vi "Edit_Channel_Panel.vi"(0 "All Channel names":string[](array[string])=["30-10-03:New:Channel new5"], 9 "Result files to read":path[](array[path]), 11 "Selected Row":i32) -> (3 "New Values Out":string[](array[string])=["Test data5"], 4 "New Chs Out":string[](array[string])=["30-10-03:New:Channel new5"], 6 "Cancel Out":bool, 8 "Edit Raw Data Header Info Out":bool, 10 "Plotted rows only?":bool, 12 "Selected Row?":bool, 13 "Edit Raw data files?":bool, 14 "Raw data files in Orig Positions?":bool, 15 "Mode":T1)   [LabVIEW 2013]
uses:
  Plotter_Mode.ctl
panel:
  out "Selected Row? 2":bool
  in  "Selected Row 2":i32
  in  "Select channel names":bool
  in  "Cancel":bool
  in  "Edit Raw data files":i32(listbox)
  in  "Columns to Output":i32[](listbox)
  in  "Edit Type":i32(listbox)
  in  "OK Button":bool
  in  "Add values to:":i32(listbox)=1
  in  "New Values In":string[](array[string])=["Value"]
  in  "New Chs In":string[](array[string])=["Channel Name"]
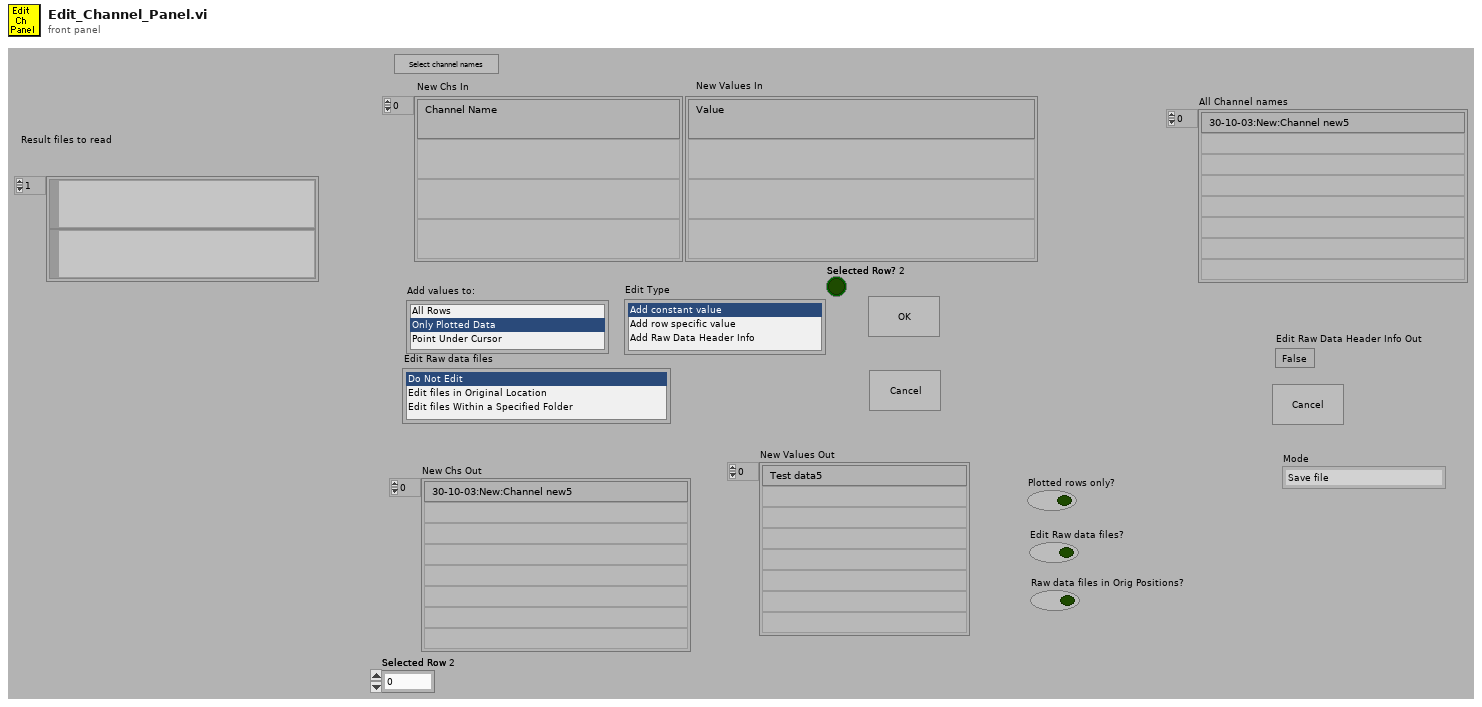
[diagram p1: front panel]
types:
  T1 = typedef "Plotter_Mode.ctl" = enum16{"Save file", "Delete unwanted rows", "Edit Values with constants", "Edit values per row", "Edit Raw Data file header", "Post Process Plotted Rows"}
  T2 = enum16{"Read Channels From File", "Read Channels from Server"}
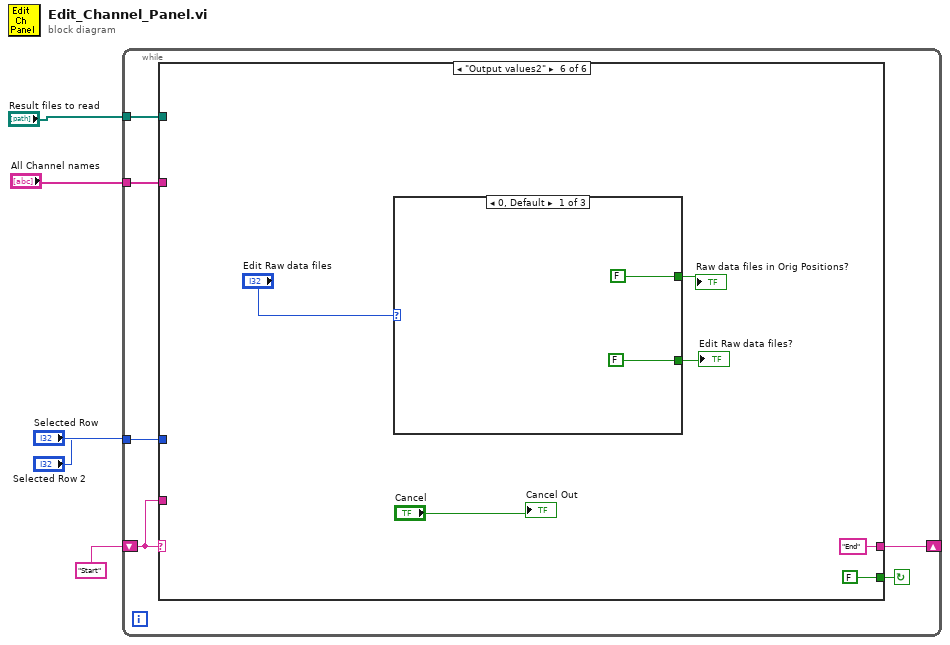
[diagram p0: block diagram]
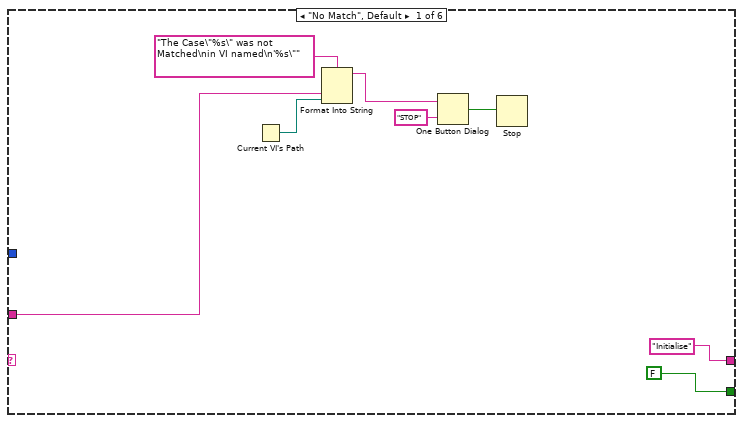
[diagram p2: hidden frame]
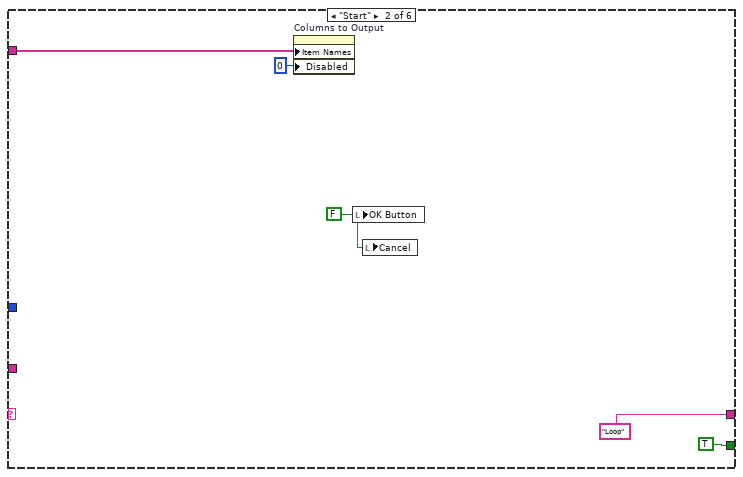
[diagram p3: hidden frame]
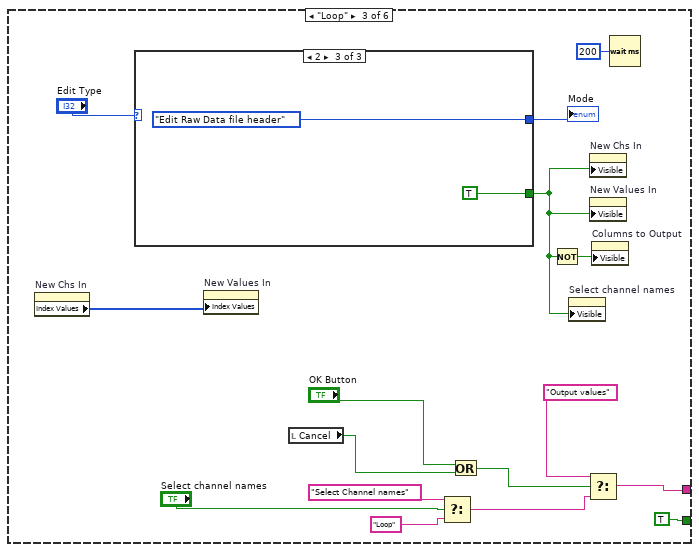
[diagram p4: hidden frame]
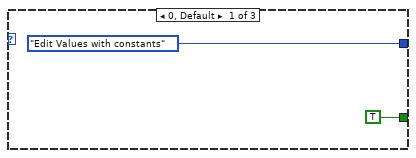
[diagram p5: hidden frame]
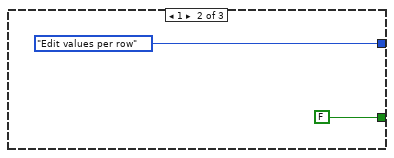
[diagram p6: hidden frame]
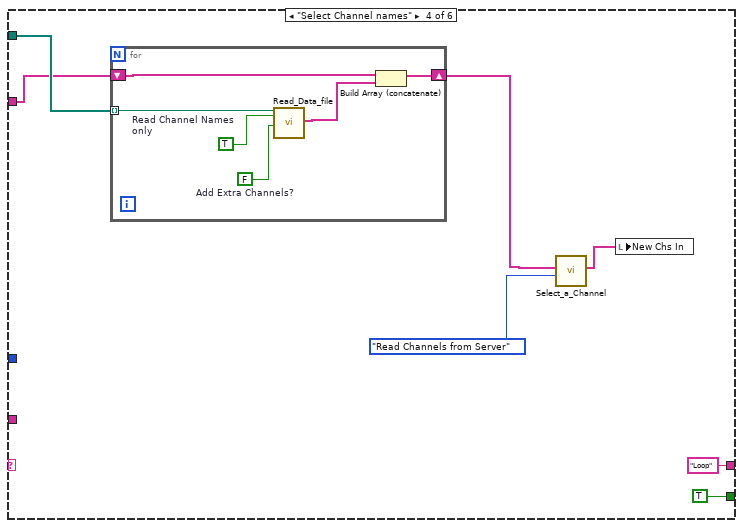
[diagram p7: hidden frame]
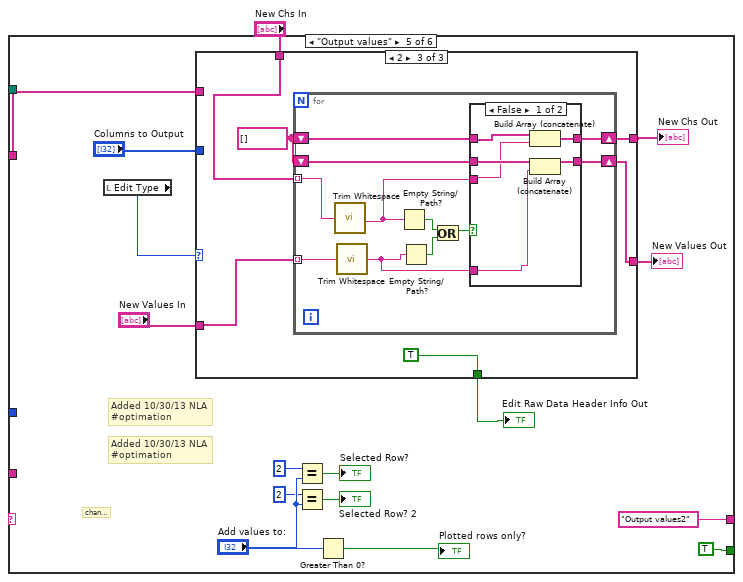
[diagram p8: hidden frame]
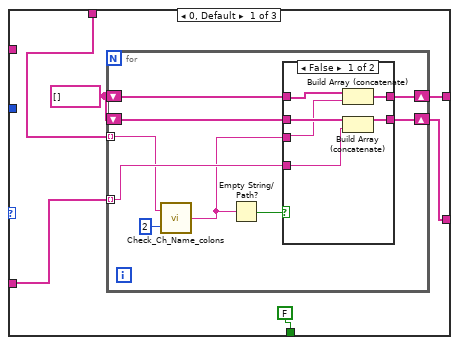
[diagram p9: hidden frame]
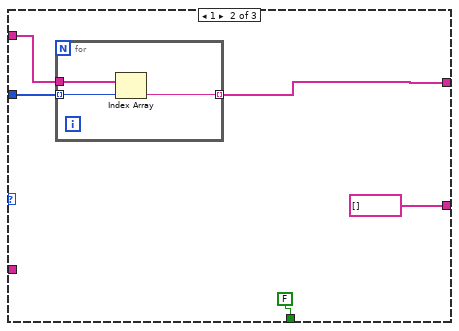
[diagram p11: hidden frame]
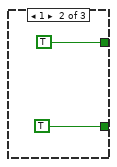
[diagram p13: hidden frame]
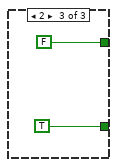
[diagram p14: hidden frame]
diagram:
  n1 = while {
    shift-left: "Start" -> [w10]
    shift-right: [w11] -> _
    tunnel: "All Channel names" -> [w9]
    tunnel: "Result files to read" -> [w8]
    tunnel: "Selected Row" -> [w7]
    tunnel: "Selected Row 2" -> [w6]
    stop <- w12 continue-if-true
    n2 = case shown="\"Output values2\"" w10 {
      tunnel: [FALSE TRUE TRUE TRUE TRUE FALSE] -> w12
      tunnel: ["Initialise" "Loop" w39 "Loop" "Output values2" "End"] -> w11
      tunnel: w10 -> [w15 _ _ _ _ _]
      tunnel: w9 -> [_ w23 _ w52 w66 _]
      tunnel: w8 -> [_ _ _ w53 _ _]
      tunnel: w7 -> [_ _ _ _ _ _]
      tunnel: w6 -> [_ _ _ _ _ _]
      frame "No Match", Default {
        n3 = Current VI's Path() -> (path=w14:path)
        n4 = Format Into String(format string="The Case\"%s\" was not Matched\nin VI named\n'%s\"" ("Format String"), w15, w14) -> (resulting string=w18:string)  [unwired: 2 in, 1 out]
        n5 = One Button Dialog(message=w18, button name ("OK")="STOP") -> (true=w16:bool)
        n6 = Stop(stop? (T)=w16) -> ()
      }
      frame "Start" {
        w21 = FALSE ("OK Button")
        n7 = property on="Columns to Output" class="LstBox (strict)"("Item Names"=w23, "Disabled"=u8 0) -> ()  [unwired: 2 in, 2 out]
        n8 = local write "OK Button"(w21) -> ()
        n9 = local write "Cancel"(w21) -> ()
      }
      frame "Loop" {
        n10 = property on="New Chs In" class="Arr (strict)"() -> ("Index Values"=w29:u32[])  [unwired: 2 in, 2 out]
        n11 = case shown="2" "Edit Type" {
          tunnel: [Plotter_Mode."Edit Values with constants" ("Mode") Plotter_Mode."Edit values per row" ("Mode") Plotter_Mode."Edit Raw Data file header" ("Mode")] -> w37
          tunnel: [TRUE FALSE TRUE] -> w26
          frame 0, Default {
          }
          frame 1 {
          }
          frame 2 {
          }
        }
        "Mode" <- w37
        n12 = property on="New Values In" class="Arr (strict)"("Index Values"=w29) -> ()  [unwired: 2 in, 2 out]
        n13 = local read "Cancel"() -> (w35:bool)
        n14 = Select(t="Select Channel names", s="Select channel names", f="Loop") -> (s? t:f=w28:string)
        n15 = Or(x="OK Button", y=w35) -> (x .or. y?=w33:bool)
        n16 = Not(x=w26) -> (.not. x?=w36:bool)
        n17 = property on="Select channel names" class="Bool"("Visible"=w26) -> ()  [unwired: 2 in, 2 out]
        n18 = Select(t="Output values", s=w33, f=w28) -> (s? t:f=w39:string)
        n19 = property on="New Chs In" class="Arr (strict)"("Visible"=w26) -> ()  [unwired: 2 in, 2 out]
        n20 = property on="New Values In" class="Arr (strict)"("Visible"=w26) -> ()  [unwired: 2 in, 2 out]
        n21 = property on="Columns to Output" class="LstBox (strict)"("Visible"=w36) -> ()  [unwired: 2 in, 2 out]
        n22 = Wait (ms)(milliseconds to wait=u32 200) -> ()  [unwired: 1 out]
      }
      frame "Select Channel names" {
        n23 = for {
          shift-right: [w57] -> w51
          shift-left: w52 -> [w55]
          tunnel: w53 -> [w60] mode=indexing
          w58 = FALSE  # Add Extra Channels?
          w59 = TRUE  # Read Channel Names only
          n24 = call "Read_Data_file.vi"("Results file"=w60, "Read Channel Names only"=w59, "Add Extra Channels?"=w58) -> ("Ch names Out"=w56:string[])  [unwired: 2 in, 14 out]
          n25 = Build Array (concatenate)(w55, w56) -> (w57:string[])
        }
        n26 = call "Select_a_Channel.vi"("Mode"=T2."Read Channels from Server", "Extra channel names"=w51) -> ("Selected Channel Names"=w50:string[])  [unwired: 1 in, 5 out]
        n27 = local write "New Chs In"(w50) -> ()
      }
      frame "Output values" {
        # "Added 10/30/13 NLA\n#optimation"
        # "Added 10/30/13 NLA\n#optimation"
        # "channel"
        n28 = local read "Edit Type"() -> (w72:i32)
        n29 = case shown="2" w72 {
          tunnel: "New Values In" -> [w80 _ w111]
          tunnel: [w79 string[] [] w110] -> w70
          tunnel: "New Chs In" -> [w81 _ w112]
          tunnel: [w78 w102 w109] -> w68
          tunnel: "Columns to Output" -> [_ w104 _]
          tunnel: w66 -> [_ w103 _]
          tunnel: [FALSE FALSE TRUE] -> w65
          frame 0, Default {
            w82 = string[] []
            n30 = for {
              tunnel: w80 -> [w87] mode=indexing
              shift-right: [w88] -> w78
              shift-left: w82 -> [w91]
              shift-right: [w90] -> w79
              shift-left: w82 -> [w89]
              tunnel: w81 -> [w86] mode=indexing
              n31 = call "Check_Ch_Name_colons.vi"("No of Colons"=2, "Ch Name in"=w86) -> ("Ch Name out"=w85:string)
              n32 = Empty String/Path?(string/path=w85) -> (empty?=w84:bool)
              n33 = case shown="False" w84 {
                tunnel: [w94 w99] -> w88
                tunnel: w91 -> [w97 w99]
                tunnel: [w95 w98] -> w90
                tunnel: w89 -> [w96 w98]
                tunnel: w87 -> [w92 _]
                tunnel: w85 -> [w93 _]
                frame False {
                  n34 = Build Array (concatenate)(w97, w93) -> (w94:string[])
                  n35 = Build Array (concatenate)(w96, w92) -> (w95:string[])
                }
                frame True {
                }
              }
            }
          }
          frame 1 {
            n36 = for {
              tunnel: w104 -> [w107] mode=indexing
              tunnel: w103 -> [w106]
              tunnel: [w105] -> w102 mode=indexing
              n37 = Index Array(array=w106, index=w107) -> (element=w105:string)
            }
          }
          frame 2 {
            w113 = string[] []
            n38 = for {
              tunnel: w111 -> [w119] mode=indexing
              shift-right: [w121] -> w109
              shift-left: w113 -> [w124]
              shift-right: [w123] -> w110
              shift-left: w113 -> [w122]
              tunnel: w112 -> [w120] mode=indexing
              n39 = call <vilib>:"Trim Whitespace.vi"("string"=w120) -> ("trimmed string"=w115:string)  [unwired: 1 in]
              n40 = call <vilib>:"Trim Whitespace.vi"("string"=w119) -> ("trimmed string"=w114:string)  [unwired: 1 in]
              n41 = Empty String/Path?(string/path=w115) -> (empty?=w117:bool)
              n42 = Empty String/Path?(string/path=w114) -> (empty?=w118:bool)
              n43 = Or(x=w117, y=w118) -> (x .or. y?=w116:bool)
              n44 = case shown="False" w116 {
                tunnel: [w127 w132] -> w121
                tunnel: w124 -> [w130 w132]
                tunnel: [w128 w131] -> w123
                tunnel: w122 -> [w129 w131]
                tunnel: w115 -> [w126 _]
                tunnel: w114 -> [w125 _]
                frame False {
                  n45 = Build Array (concatenate)(w130, w126) -> (w127:string[])
                  n46 = Build Array (concatenate)(w129, w125) -> (w128:string[])
                }
                frame True {
                }
              }
            }
          }
        }
        "New Values Out" <- w70
        "New Chs Out" <- w68
        "Edit Raw Data Header Info Out" <- w65
        n47 = Equal?(x=2, y="Add values to:") -> (x = y?=→"Selected Row?":bool)
        n48 = Equal?(x=2, y="Add values to:") -> (x = y?=→"Selected Row? 2":bool)
        n49 = Greater Than 0?(x="Add values to:") -> (x > 0?=→"Plotted rows only?":bool)
      }
      frame "Output values2" {
        n50 = case shown="0, Default" "Edit Raw data files" {
          tunnel: [FALSE TRUE TRUE] -> w135
          tunnel: [FALSE TRUE FALSE] -> w134
          frame 0, Default {
          }
          frame 1 {
          }
          frame 2 {
          }
        }
        "Edit Raw data files?" <- w135
        "Raw data files in Orig Positions?" <- w134
        "Cancel Out" <- "Cancel"
      }
    }
  }
